vi "Action Start Pump.vi"(5 "Retry Attempts (0)":i32 min=0, 8 "error in":errorcluster, 11 "VISA resource name":refnum<visa-resource-name>) -> (0 "error out":errorcluster, 3 "VISA resource name out":refnum<visa-resource-name>)   [LabVIEW 2020, in "ChromTech Series III Pump.lvlib"]
doc: "Run the pump."
uses:
  <instrlib>/RxnRover/ChromtechSeriesIIIDriver/ChromTech Series III Pump.lvlib
panel:
  out "Response":string
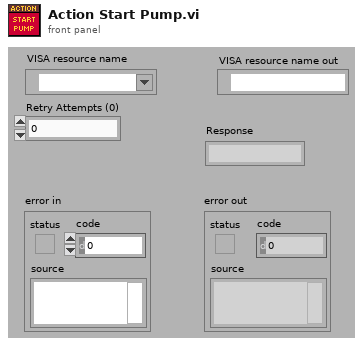
[diagram p1: front panel]
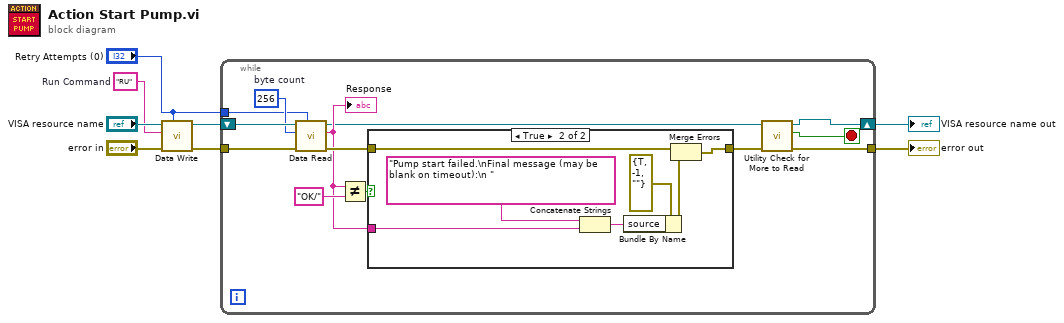
[diagram p0: block diagram]
diagram:
  w5 = "RU"  # Run Command
  n1 = call <instrlib>:"Data Write.vi"("Retry Attempts (0)"="Retry Attempts (0)", "error in (no error)"="error in", "Command"=w5, "VISA Refnum in"="VISA resource name") -> ("error out"=w3:errorcluster, "VISA Refnum out"=w7:refnum<visa-resource-name>)  [unwired: 6 in]
  n2 = while {
    shift-right: [w12] -> w4
    shift-left: w7 -> [w21]
    tunnel: "Retry Attempts (0)" -> [w14]
    tunnel: w3 -> [w17]
    tunnel: [w10] -> w2
    stop <- w9 stop-if-true
    w20 = u32 256  # byte count
    n3 = call <instrlib>:"Data Read.vi"("Retry Attempts (0)"=w14, "error in (no error)"=w17, "Bytes to read"=w20, "VISA Refnum in"=w21) -> ("error out"=w16:errorcluster, "read buffer"=w15:string, "VISA Refnum out"=w13:refnum<visa-resource-name>)  [unwired: 5 in]
    "Response" <- w15
    n4 = Not Equal?(x=w15, y="OK/") -> (x != y?=w18:bool)
    n5 = case shown="True" w18 {
      tunnel: [w22 w28] -> w11
      tunnel: w16 -> [w22 w27]
      tunnel: w15 -> [_ w23]
      frame False {
      }
      frame True {
        n6 = Concatenate Strings("Pump start failed.\nFinal message (may be blank on timeout):\n ", w23) -> (w25:string)
        n7 = Bundle By Name(cluster=errorcluster {"status"=TRUE, "code"=-1, "source"=""} ("error out"), "source"=w25) -> (w26:errorcluster)
        n8 = Merge Errors(w27, w26) -> (w28:errorcluster)
      }
    }
    n9 = call <instrlib>:"Utility Check for More to Read.vi"("error in (no error)"=w11, "VISA Refnum in"=w13) -> ("error out (unchanged)"=w10:errorcluster, "More to read?"=w9:bool, "VISA Refnum out"=w12:refnum<visa-resource-name>)  [unwired: 7 in]
  }
  "VISA resource name out" <- w4
  "error out" <- w2
